vi "LM Gaussian and gradient.vi"(3 "output control":T1, 4 "data":variant, 5 "X":dbl[](array[numeric]), 6 "a":dbl[](array[numeric])) -> (0 "error out":errorcluster, 1 "f'(X,a)":dbl[][](array[numeric]), 2 "f(X,a)":dbl[](array[numeric]))   [LabVIEW 2021, in "Fits.lvlib"]
doc: "This template is the starting point for creating a model function to be passed to the Nonlinear Curve Fit.vi."
uses:
  <vilib>/gmath/NumericalOptimization/LM_output select.ctl
  Fits.lvlib
  <vilib>/gmath/NI_Gmath.lvlib
panel:
  # "Parameters:\n\namplitude: A\ncenter: x_0\nSDV: s"
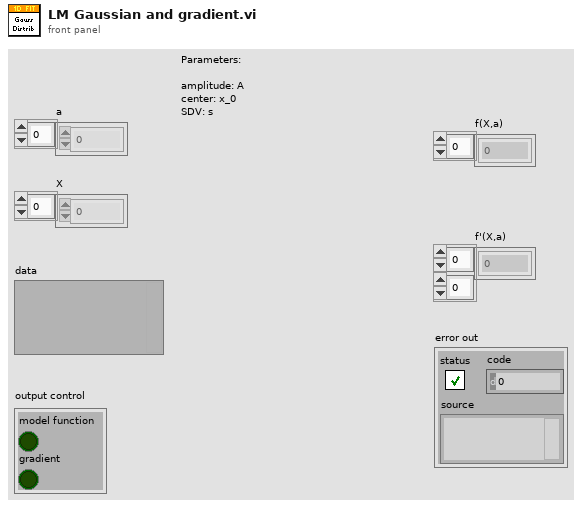
[diagram p1: front panel]
types:
  T1 = typedef "NI_Gmath.lvlib/LM_output select.ctl" = cluster{"model function":bool, "gradient":bool}
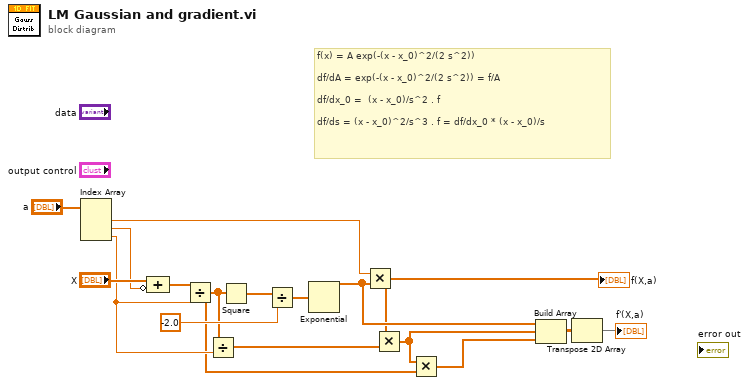
[diagram p0: block diagram]
diagram:
  # "f(x) = A exp(-(x - x_0)^2/(2 s^2))\n\ndf/dA = exp(-(x - x_0)^2/(2 s^2)) = f/A\n\ndf/dx_0 =  (x - x_0)/s^2 . f\n\ndf/ds = (x - x_0)^2/s^3 . f = df/dx_0 * (x - x_0)/s"
  n1 = Index Array(array="a") -> (element #1=w10:dbl, element #2=w15:dbl, element #3=w9:dbl)  [unwired: 3 in]
  n2 = Compound Arithmetic op=ADD("X", invert w15) -> (w14:dbl[])
  n3 = Divide(x=w14, y=w9) -> (x/y=w4:dbl[])
  n4 = Divide(x=w4, y=w9) -> (x/y=w6:dbl[])
  n5 = Square(x=w4) -> (x^2=w12:dbl[])
  n6 = Divide(x=w12, y=-2.0 ("element")) -> (x/y=w11:dbl[])
  n7 = Exponential(1:w11) -> (0:w8:dbl[])
  n8 = Multiply(x=w10, y=w8) -> (x*y=w7:dbl[])
  "f(X,a)" <- w7
  n9 = Multiply(x=w7, y=w6) -> (x*y=w5:dbl[])
  n10 = Multiply(x=w5, y=w4) -> (x*y=w3:dbl[])
  n11 = Build Array(w8, w5, w3) -> (w2:dbl[][])
  n12 = Transpose 2D Array(2D array=w2) -> (transposed array=→"f'(X,a)":dbl[][])
